vi "custom_email_program.vi"(5 "mail server":string="smtp.nikhef.nl", 7 "return address":string="xamsups@gmail.com", 8 "error in (no error)":errorcluster, 9 "message":string, 10 "subject ([No Subject])":string="[No Subject]", 11 "Email Adresses":string[](array[string])) -> (0 "error out":errorcluster)   [LabVIEW 2018]
uses:
  <vilib>/Utility/SMTP/NI_SMTPEmail.lvlib
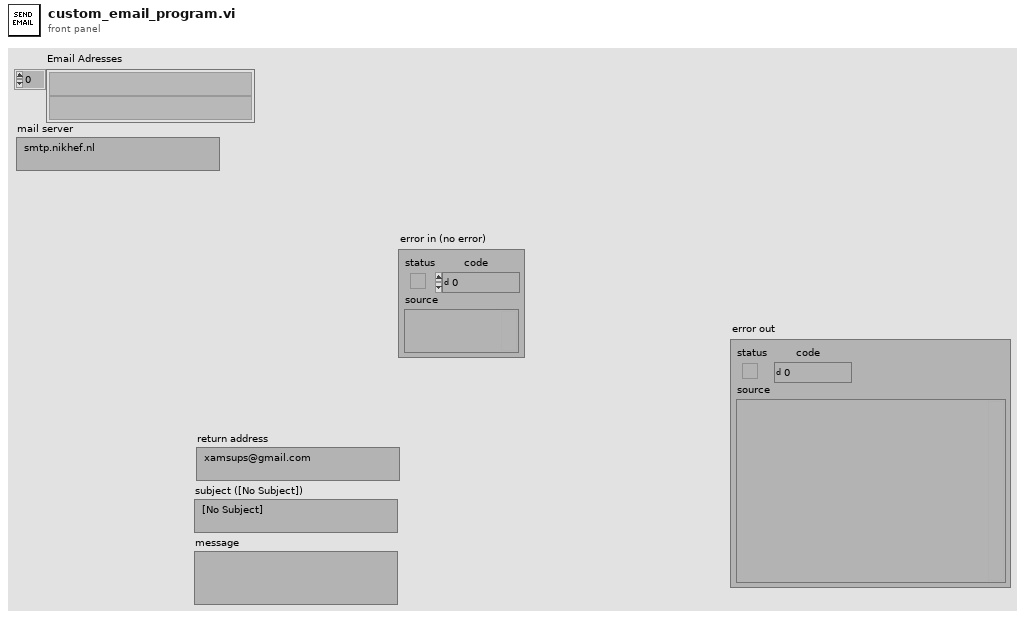
[diagram p1: front panel]
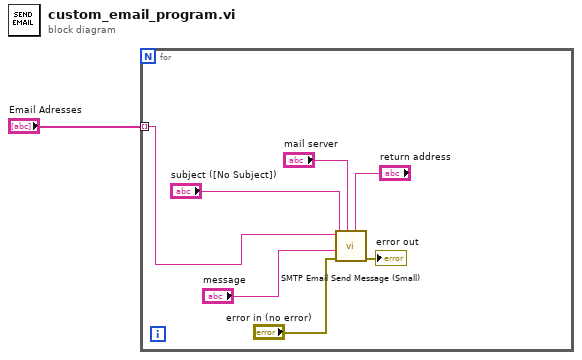
[diagram p0: block diagram]
diagram:
  n1 = for {
    tunnel: "Email Adresses" -> [w3] mode=indexing
    n2 = call <vilib>:"SMTP Email Send Message (Small).vi"("return address"="return address", "mail server"="mail server", "error in (no error)"="error in (no error)", "message"="message", "subject ([No Subject])"="subject ([No Subject])", "recipient"=w3) -> ("error out"=→"error out":errorcluster)  [unwired: 5 in]
  }
